vi "Tear Down.vi"(8 "error in (no error)":errorcluster, 11 "Assembler in":refnum<class "Assembler.lvclass">) -> (0 "error out":errorcluster, 3 "Assembler out":refnum<class "Assembler.lvclass">)   [LabVIEW 2016, in "CLD Exam - ATM.lvlib" / "Assembler.lvclass"]
uses:
  Assembler.lvclass
  Assembler.lvclass/Assembler.ctl
  User Interface/User Interface.lvclass
  Terminal Timeout/Terminal Timeout.lvclass
  Terminal Menus/Terminal Menus.lvclass
  Terminal Message/Terminal Message.lvclass
  Bank Account/Bank Account.lvclass
  Replay/Replay.lvclass
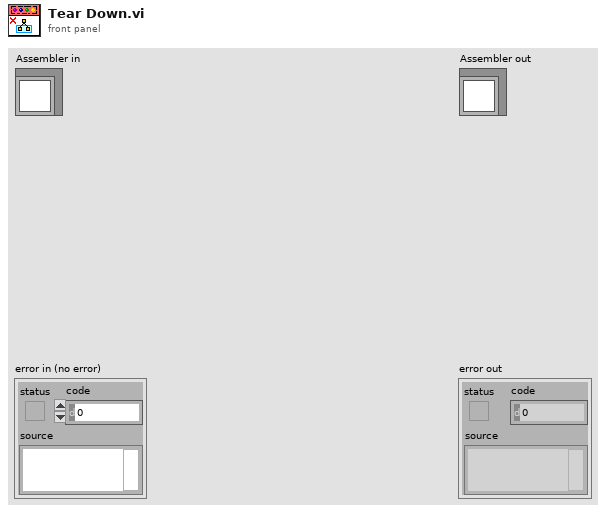
[diagram p1: front panel]
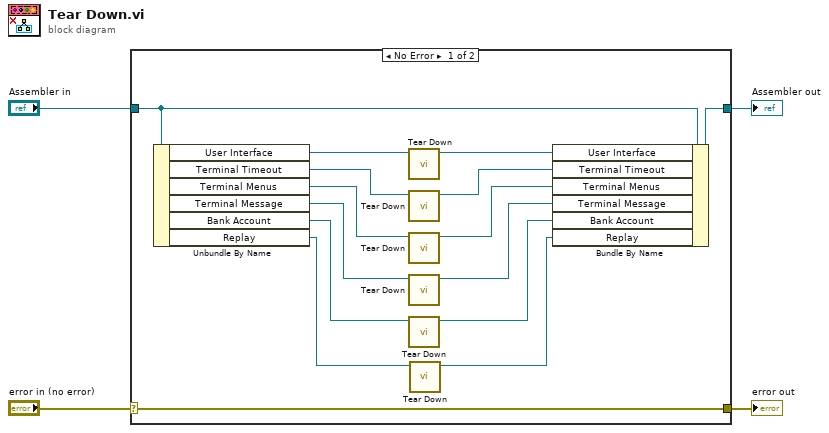
[diagram p0: block diagram]
diagram:
  n1 = case shown="No Error" "error in (no error)" {
    selector: "error in (no error)" -> [w19 w21]
    tunnel: [w19 w21] -> w3
    tunnel: [w15 w20] -> w1
    tunnel: "Assembler in" -> [w16 w20]
    frame No Error {
      n2 = Unbundle By Name(w16) -> ("User Interface"=w18:refnum<class "User Interface.lvclass">, "Terminal Timeout"=w14:refnum<class "Terminal Timeout.lvclass">, "Terminal Menus"=w12:refnum<class "Terminal Menus.lvclass">, "Terminal Message"=w10:refnum<class "Terminal Message.lvclass">, "Bank Account"=w8:refnum<class "Bank Account.lvclass">, "Replay"=w6:refnum<class "Replay.lvclass">)
      n3 = call "Tear Down.vi"("User Interface in"=w18) -> ("User Interface out"=w17:refnum<class "User Interface.lvclass">)  [unwired: 9 in, 1 out]
      n4 = call "Tear Down.vi"("Terminal Timeout in"=w14) -> ("Terminal Timeout out"=w13:refnum<class "Terminal Timeout.lvclass">)  [unwired: 9 in, 1 out]
      n5 = call "Tear Down.vi"("Terminal Menus in"=w12) -> ("Terminal Menus out"=w11:refnum<class "Terminal Menus.lvclass">)  [unwired: 9 in, 1 out]
      n6 = call "Tear Down.vi"("Terminal Message in"=w10) -> ("Terminal Message out"=w9:refnum<class "Terminal Message.lvclass">)  [unwired: 9 in, 1 out]
      n7 = call "Tear Down.vi"("Bank Account in"=w8) -> ("Bank Account out"=w7:refnum<class "Bank Account.lvclass">)  [unwired: 9 in, 1 out]
      n8 = call "Tear Down.vi"("Replay in"=w6) -> ("Replay out"=w5:refnum<class "Replay.lvclass">)  [unwired: 9 in, 1 out]
      n9 = Bundle By Name(cluster=w16, "User Interface"=w17, "Terminal Timeout"=w13, "Terminal Menus"=w11, "Terminal Message"=w9, "Bank Account"=w7, "Replay"=w5) -> (w15:refnum<class "Assembler.lvclass">)
    }
    frame Error {
    }
  }
  "error out" <- w3
  "Assembler out" <- w1
